vi "Update proto text.vi"(8 "error in":errorcluster, 10 "New Subname":string, 11 "Proto Text In":string) -> (0 "error out":errorcluster, 1 "snake_case":string, 2 "gRPC Service Name":string, 3 "Proto Text Out":string)   [LabVIEW 2021, in "Plugin Generator.lvlib"]
uses:
  Plugin Generator.lvlib
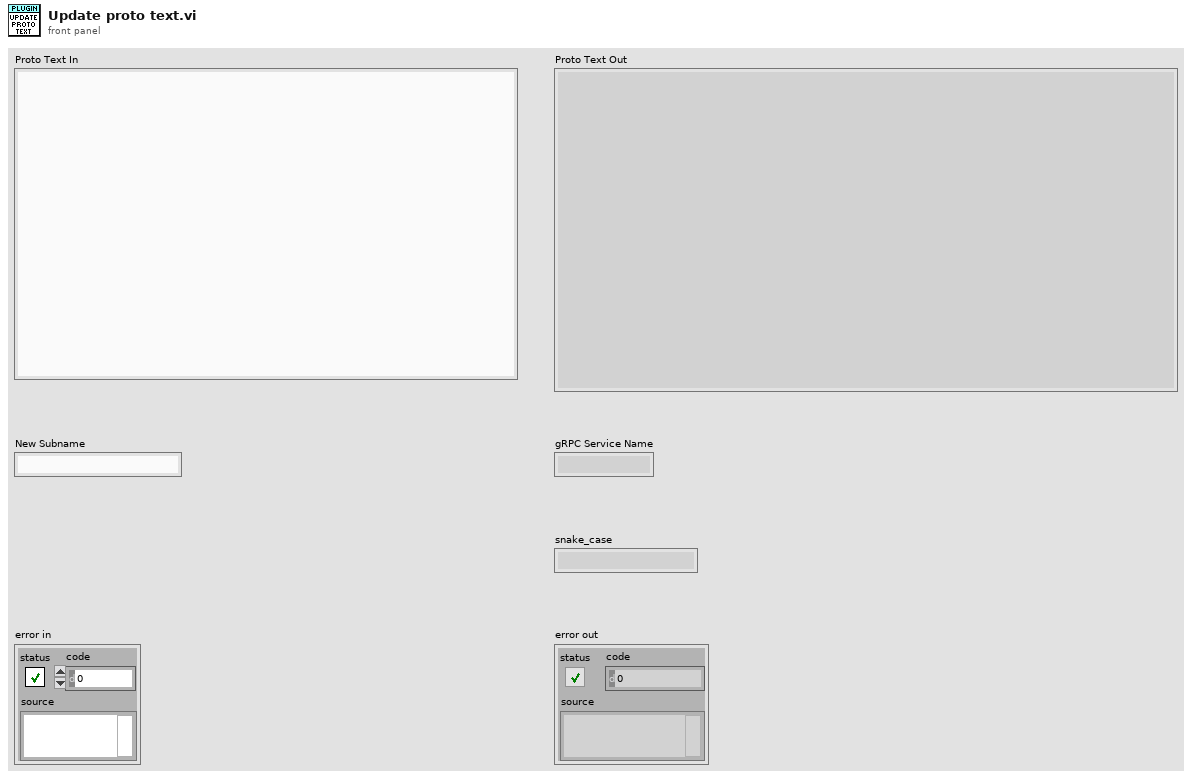
[diagram p1: front panel]
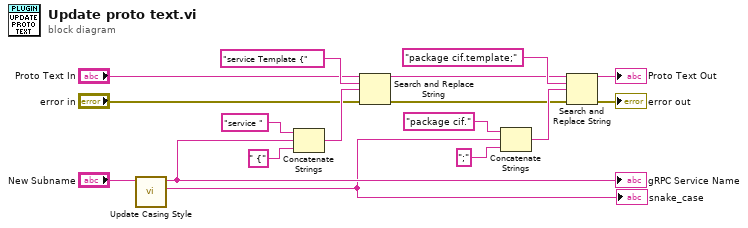
[diagram p0: block diagram]
diagram:
  n1 = call "Update Casing Style.vi"("Input Name"="New Subname") -> ("snake_case"=w3:string, "PascalCase"=w12:string)  [unwired: 9 in]
  "gRPC Service Name" <- w12
  "snake_case" <- w3
  n2 = Concatenate Strings("service ", w12, " {") -> (w16:string)
  n3 = Search and Replace String(input string="Proto Text In", search string="service Template {", replace string=w16, error in="error in") -> (result string=w5:string, error out=w4:errorcluster)  [unwired: 4 in, 2 out]
  n4 = Concatenate Strings("package cif.", w3, ";") -> (w6:string)
  n5 = Search and Replace String(input string=w5, search string="package cif.template;", replace string=w6, error in=w4) -> (result string=→"Proto Text Out":string, error out=→"error out":errorcluster)  [unwired: 4 in, 2 out]
